vi "consec.vi"(1 "String":string, 2 "Start":i32, 3 "Array":cluster{string, "number of columns":i32}[](array[cluster])) -> (0 "Numeric":i32)   [LabVIEW 2019]
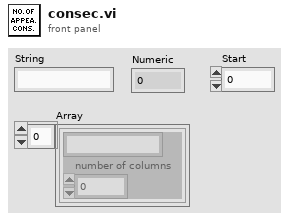
[diagram p1: front panel]
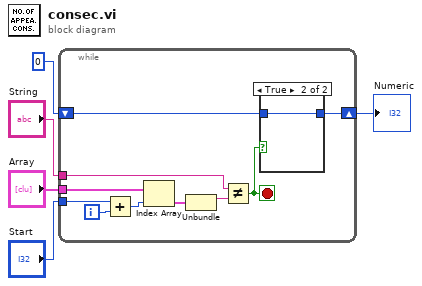
[diagram p0: block diagram]
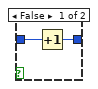
[diagram p2: hidden frame]
diagram:
  n1 = while {
    tunnel: "Start" -> [w14]
    tunnel: "Array" -> [w12]
    tunnel: "String" -> [w9]
    shift-right: [w6] -> w2
    shift-left: 0 -> [w7]
    i -> [w15]
    stop <- w8 stop-if-true
    n2 = Add(x=w14, y=w15) -> (x+y=w13:i32)
    n3 = Index Array(array=w12, index=w13) -> (element=w11:cluster{string, "number of columns":i32})
    n4 = Unbundle(w11) -> (w10:string)  [unwired: 1 out]
    n5 = Not Equal?(x=w9, y=w10) -> (x != y?=w8:bool)
    n6 = case shown="True" w8 {
      tunnel: w7 -> [w17 w18]
      tunnel: [w16 w18] -> w6
      frame False {
        n7 = Increment(x=w17) -> (x+1=w16:i32)
      }
      frame True {
      }
    }
  }
  "Numeric" <- w2
